vi "Read Stop Module Loop.vi"(11 "Module Ident":string) -> (2 "error out":errorcluster, 3 "Stop":bool, 5 "notifier out":refnum<notifier>)   [LabVIEW 2024]
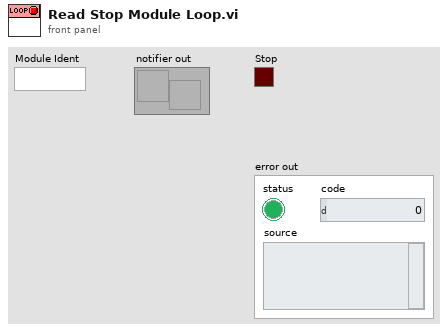
[diagram p1: front panel]
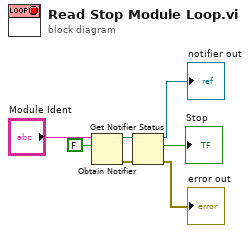
[diagram p0: block diagram]
diagram:
  n1 = Obtain Notifier(name (unnamed)="Module Ident", notification data type=FALSE) -> (notifier out=w4:refnum<notifier>, error out=w3:errorcluster)  [unwired: 2 in, 1 out]
  n2 = Get Notifier Status(notifier=w4, error in (no error)=w3) -> (notifier out=→"notifier out":refnum<notifier>, current notification=→"Stop":bool, error out=→"error out":errorcluster)  [unwired: 2 out]
